vi "Create Save Plot Grid.vi"() -> ()   [LabVIEW 2013]
uses:
  Controls/Type of Neuron.ctl
  <vilib>/Utility/miscctls.llb/LV3DPointTypeDef.ctl
  <vilib>/Analysis/coordinate.llb/3D Coordinate Conversion (Scalar).vi
  <vilib>/Analysis/NI_AALPro.lvlib
  Cube/Grid.lvclass
panel:
  out "Allocating":dbl(slide) scale=0.0..1.0
  out "No Neurons":i32=343
  out "error out":errorcluster
  in  "stop":bool
  in  "Camera Position":cluster{"X":sgl, "Y":sgl, "Z":sgl}={"X"=0.0, "Y"=250.0, "Z"=100.0}
  out "3D Picture":refnum<vi>(3d-picture)
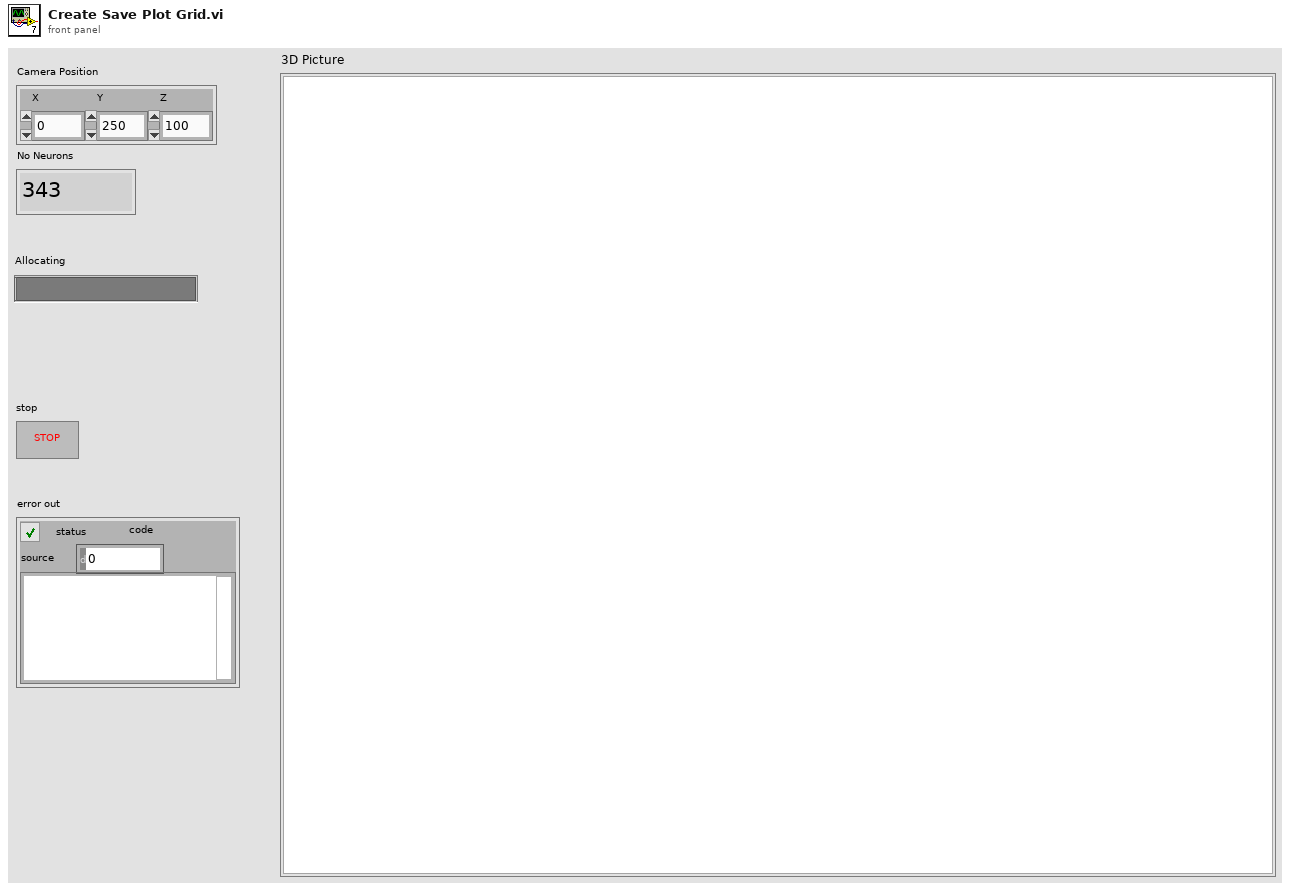
[diagram p1: front panel]
types:
  T1 = typedef "Type of Neuron.ctl" = enum16{"MF", "BA", "GO", "GC", "PC", "LU", "Glia (Dummy)"}
  T2 = typedef "LV3DPointTypeDef.ctl" = cluster{"X":sgl, "Y":sgl, "Z":sgl}
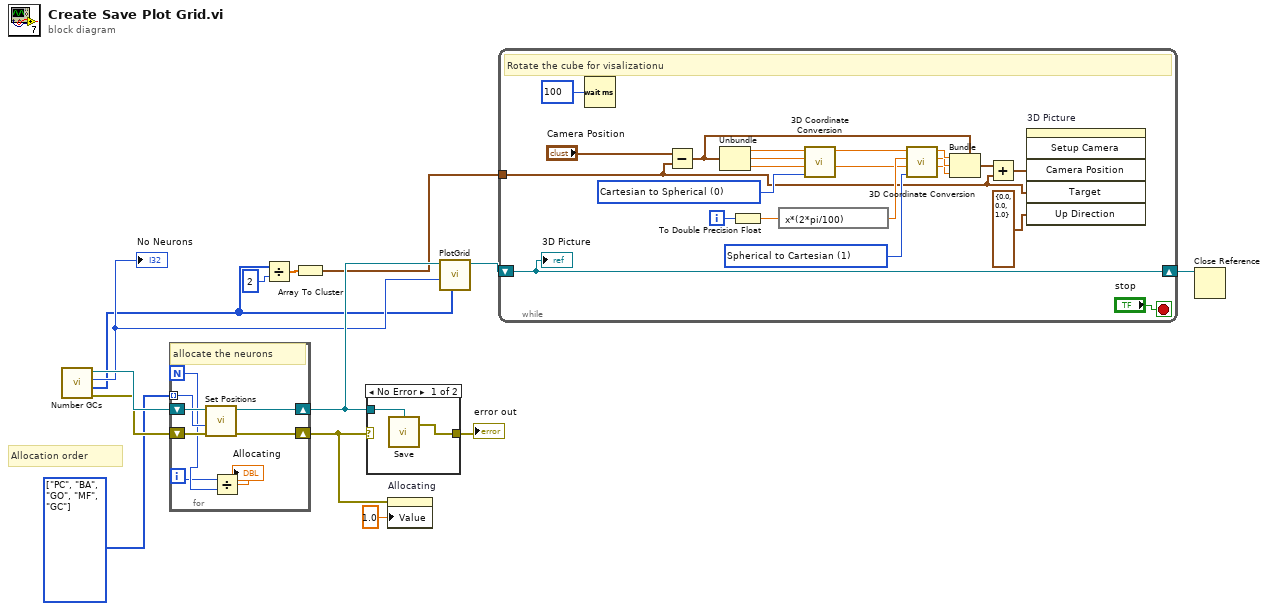
[diagram p0: block diagram]
diagram:
  w3 = T1[] [enum."PC", enum."BA", enum."GO", enum."MF", enum."GC"] items=["MF", "BA", "GO", "GC", "PC", "LU", "Glia (Dummy)"]
  # "Allocation order"
  n1 = call "Number GCs.vi"() -> ("error out"=w6:errorcluster, "Size (um)"=w8:u32[], "No Total Neurons"=w9:i32, "Cube out"=w13:refnum<class "Grid.lvclass">)  [unwired: 5 in]
  "No Neurons" <- w9
  n2 = for {
    N -> [w17]
    shift-right: [w21] -> w10
    shift-left: w13 -> [w22]
    tunnel: w3 -> [w18] mode=indexing
    shift-right: [w20] -> w2
    shift-left: w6 -> [w19]
    i -> [w15]
    # "allocate the neurons"
    n3 = call "Set Positions.vi"("error in"=w19, "Type of Neuron"=w18, "Grid in"=w22) -> ("error out"=w20:errorcluster, "Grid out"=w21:refnum<class "Grid.lvclass">)  [unwired: 7 in]
    n4 = Divide(x=w15, y=w17) -> (x/y=→"Allocating":dbl)
  }
  n5 = Divide(x=w8, y=2 ("Numeric")) -> (x/y=w5:dbl[])
  n6 = Array To Cluster(array=w5) -> (cluster=w4:cluster{"[0]":dbl, "[1]":dbl, "[2]":dbl})
  n7 = case shown="No Error" w2 {
    selector: w2 -> [_ w25]
    tunnel: w10 -> [w24 _]
    tunnel: [w23 w25] -> w7
    frame No Error {
      n8 = call "Save.vi"("Grid in"=w24) -> ("error out"=w23:errorcluster)  [unwired: 1 in, 1 out]
    }
    frame Error {
    }
  }
  "error out" <- w7
  n9 = property on="Allocating" class="Slide (strict)"(error in=w2, "Value"=1.0 ("Allocating")) -> ()  [unwired: 1 in, 2 out]
  n10 = call "PlotGrid.vi"("Size (um)"=w8, "No Neurons"=w9, "Grid in"=w10) -> ("Scene Object Out"=w12:refnum<vi>)  [unwired: 8 in]
  n11 = while {
    shift-right: [w47] -> w11
    shift-left: w12 -> [w47]
    tunnel: w4 -> [w26]
    i -> [w42]
    stop <- "stop" stop-if-true
    w39 = u16 1 items=["Cartesian to Spherical", "Spherical to Cartesian", "Cartesian to Cylindrical", "Cylindrical to Cartesian", "Spherical to Cylindrical", "Cylindrical to Spherical"] ("conversion type")
    w43 = u16 0 items=["Cartesian to Spherical", "Spherical to Cartesian", "Cartesian to Cylindrical", "Cylindrical to Cartesian", "Spherical to Cylindrical", "Cylindrical to Spherical"] ("conversion type")
    # "Rotate the cube for visalizationu"
    n12 = Wait (ms)(milliseconds to wait=u32 100) -> ()  [unwired: 1 out]
    n13 = Subtract(x="Camera Position", y=w26) -> (x-y=w29:cluster{dbl, dbl, dbl})
    n14 = Unbundle(w29) -> (w46:dbl, w45:dbl, w44:dbl)
    n15 = To Double Precision Float(number=w42) -> (double precision float=w41:dbl)
    n16 = expression code="x*(2*pi/100)"(w41) -> (w32:dbl)
    n17 = call-poly <vilib>:"3D Coordinate Conversion.vi"("conversion type"=w43, "axis 3"=w44, "axis 2"=w45, "axis 1"=w46) -> ("axis 3 out"=w31:dbl, "axis 1 out"=w40:dbl)  [unwired: 4 in, 2 out]
    n18 = call-poly <vilib>:"3D Coordinate Conversion.vi"("conversion type"=w39, "axis 3"=w31, "axis 2"=w32, "axis 1"=w40) -> ("axis 3 out"=w36:dbl, "axis 2 out"=w37:dbl, "axis 1 out"=w38:dbl)  [unwired: 4 in, 1 out]
    n19 = Bundle(cluster=w29, w38, w37, w36) -> (w28:cluster{dbl, dbl, dbl})
    n20 = Add(x=w28, y=w26) -> (x+y=w27:cluster{dbl, dbl, dbl})
    n21 = invoke on="3D Picture" class="SceneGraphDisp (strict)" method="Setup Camera"("Camera Position"=w27, "Target"=w26, "Up Direction"=T2 {"X"=0.0, "Y"=0.0, "Z"=1.0}) -> ()  [unwired: 3 in, 6 out]
    "3D Picture" <- w47
  }
  n22 = Close Reference(reference=w11) -> ()  [unwired: 1 in, 1 out]
